vi "Write RampArray.vi"(8 "error in (no error)":errorcluster, 11 "RampProgramModel in":refnum<class "RampProgramModel.lvclass">) -> (0 "error out":errorcluster, 3 "RampProgramModel out":refnum<class "RampProgramModel.lvclass">)   [LabVIEW 2013, in "RampProgramModel.lvclass"]
uses:
  RampProgramModel.lvclass
  RampProgramModel.lvclass/RampProgramModel.ctl
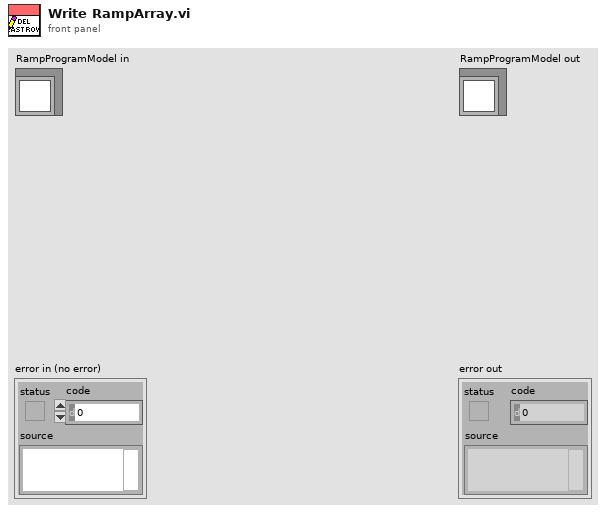
[diagram p1: front panel]
types:
  T1 = cluster{"SP (°C)":dbl, "Cooling rate (°C/min)":dbl, "Dwell Time @ SP (sec)":u32}[]
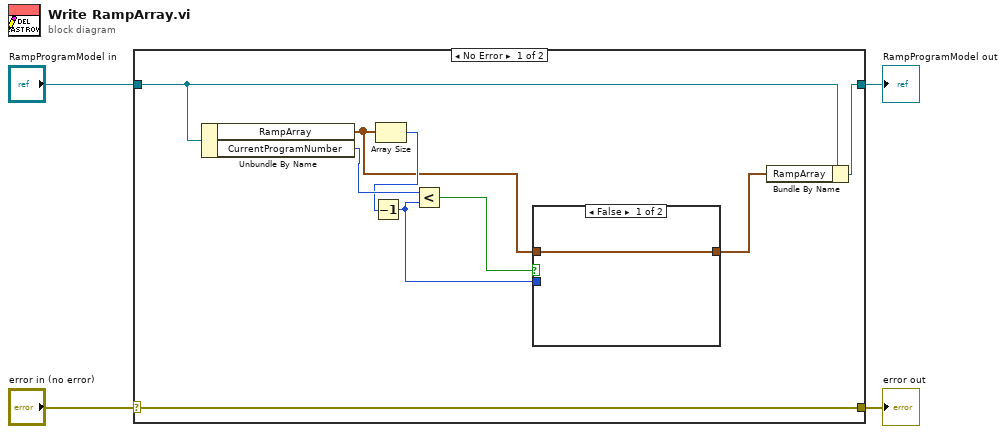
[diagram p0: block diagram]
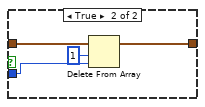
[diagram p2: hidden frame]
diagram:
  n1 = case shown="No Error" "error in (no error)" {
    selector: "error in (no error)" -> [w13 w19]
    tunnel: [w13 w19] -> w3
    tunnel: [w12 w20] -> w1
    tunnel: "RampProgramModel in" -> [w11 w20]
    frame No Error {
      n2 = Unbundle By Name(w11) -> ("RampArray"=w7:T1, "CurrentProgramNumber"=w10:u32)
      n3 = Array Size(array=w7) -> (size(s)=w9:i32)
      n4 = Decrement(x=w9) -> (x-1=w6:i32)
      n5 = Less?(x=w10, y=w6) -> (x < y?=w8:bool)
      n6 = case shown="False" w8 {
        tunnel: w7 -> [w14 w18]
        tunnel: w6 -> [_ w17]
        tunnel: [w14 w15] -> w5
        frame False {
        }
        frame True {
          n7 = Delete From Array(array=w18, length=1, index=w17) -> (array with subset deleted=w15:T1)  [unwired: 1 out]
        }
      }
      n8 = Bundle By Name(cluster=w11, "RampArray"=w5) -> (w12:refnum<class "RampProgramModel.lvclass">)
    }
    frame Error {
    }
  }
  "error out" <- w3
  "RampProgramModel out" <- w1
